vi "Ramp PSU to Target X.vi"(8 "error in (no error)":errorcluster, 9 "Target Rate (T/min)":dbl, 10 "Target Field (T)":dbl, 11 "Instrument.OxfordVRM in":refnum<class "Instrument.OxfordVRM.lvclass">) -> (0 "error out":errorcluster, 3 "Instrument.OxfordVRM out":refnum<class "Instrument.OxfordVRM.lvclass">)   [LabVIEW 2016, in "Instrument.OxfordVRM.lvclass"]
uses:
  Instrument.OxfordVRM.lvclass
  <instrlib>/Mercury iXX/Public/Libraries/Magnet/Controls/PSU Actions.ctl
  <instrlib>/Mercury iXX/Public/Libraries/Magnet.lvlib
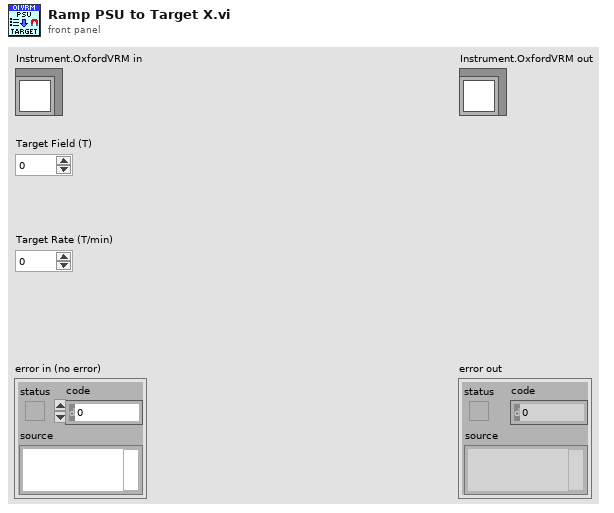
[diagram p1: front panel]
types:
  T1 = typedef "Mercury iXX.lvlib/Magnet.lvlib/PSU Actions.ctl" = string
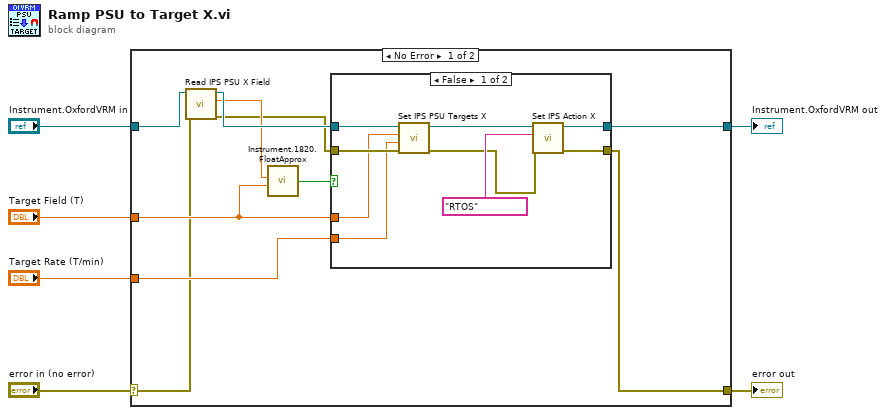
[diagram p0: block diagram]
diagram:
  n1 = case shown="No Error" "error in (no error)" {
    selector: "error in (no error)" -> [w11 w29]
    tunnel: [w7 w29] -> w5
    tunnel: [w16 w28] -> w3
    tunnel: "Instrument.OxfordVRM in" -> [w12 w28]
    tunnel: "Target Field (T)" -> [w14 _]
    tunnel: "Target Rate (T/min)" -> [w13 _]
    frame No Error {
      n2 = call "Read IPS PSU X Field.vi"("error in (no error)"=w11, "Instrument.OxfordVRM in"=w12) -> ("error out"=w8:errorcluster, "Power Supply Field (T)"=w9:dbl, "Instrument.OxfordVRM out"=w10:refnum<class "Instrument.OxfordVRM.lvclass">)  [unwired: 7 in]
      n3 = call "Instrument.1820.FloatApprox.vi"("y"=w14, "x"=w9) -> ("x ~ y?"=w15:bool)  [unwired: 4 in]
      n4 = case shown="False" w15 {
        tunnel: [w17 w27] -> w16
        tunnel: [w18 w26] -> w7
        tunnel: w10 -> [w22 w27]
        tunnel: w8 -> [w25 w26]
        tunnel: w14 -> [w23 _]
        tunnel: w13 -> [w24 _]
        frame False {
          n5 = call "Set IPS PSU Targets X.vi"("error in (no error)"=w25, "Target Field Rate (T/min)"=w24, "Target Field (T)"=w23, "Instrument.OxfordVRM in"=w22) -> ("error out"=w19:errorcluster, "Instrument.OxfordVRM out"=w21:refnum<class "Instrument.OxfordVRM.lvclass">)  [unwired: 5 in, 1 out]
          n6 = call "Set IPS Action X.vi"("error in (no error)"=w19, "PSU Act Stat"=T1 "RTOS", "Instrument.OxfordVRM in"=w21) -> ("error out"=w18:errorcluster, "Instrument.OxfordVRM out"=w17:refnum<class "Instrument.OxfordVRM.lvclass">)  [unwired: 6 in, 1 out]
        }
        frame True {
          # "If PSU Field == Target, do nothing"
        }
      }
    }
    frame Error {
    }
  }
  "error out" <- w5
  "Instrument.OxfordVRM out" <- w3
